vi "应用举例（按位反转加密解密）.vi"() -> ()   [LabVIEW 2012]
panel:
  out "加密字符串":string
  out "解密字符串":string
  in  "输入字符串":string
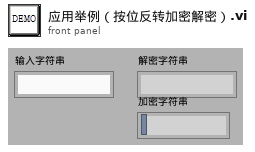
[diagram p1: front panel]
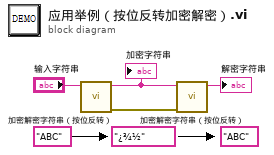
[diagram p0: block diagram]
diagram:
  (unwired) "ABC" ("解密字符串")
  (unwired) "¿¾½" ("加密字符串")
  (unwired) "ABC" ("输入字符串")
  n1 = call "加密解密字符串（按位反转）.vi"("输入字符串"="输入字符串") -> ("error out"=w3:errorcluster, "加密字符串"=w2:string)  [unwired: 9 in]
  "加密字符串" <- w2
  n2 = call "加密解密字符串（按位反转）.vi"("error in (no error)"=w3, "输入字符串"=w2) -> ("加密字符串"=→"解密字符串":string)  [unwired: 8 in, 1 out]
